vi "gmmregRegistrationTestNew.vi"() -> ()   [LabVIEW 2017]
panel:
  out "optogenetics (scene)":dbl[][](array[numeric])
  out "XY Graph 4":cluster{dbl[], dbl[]}[](graph)
  out "XY Graph 3":cluster{dbl[], dbl[]}(graph)
  out "XY Graph 2":cluster{dbl[], dbl[]}[](graph)
  out "XY Graph":cluster{dbl[], dbl[]}(graph)
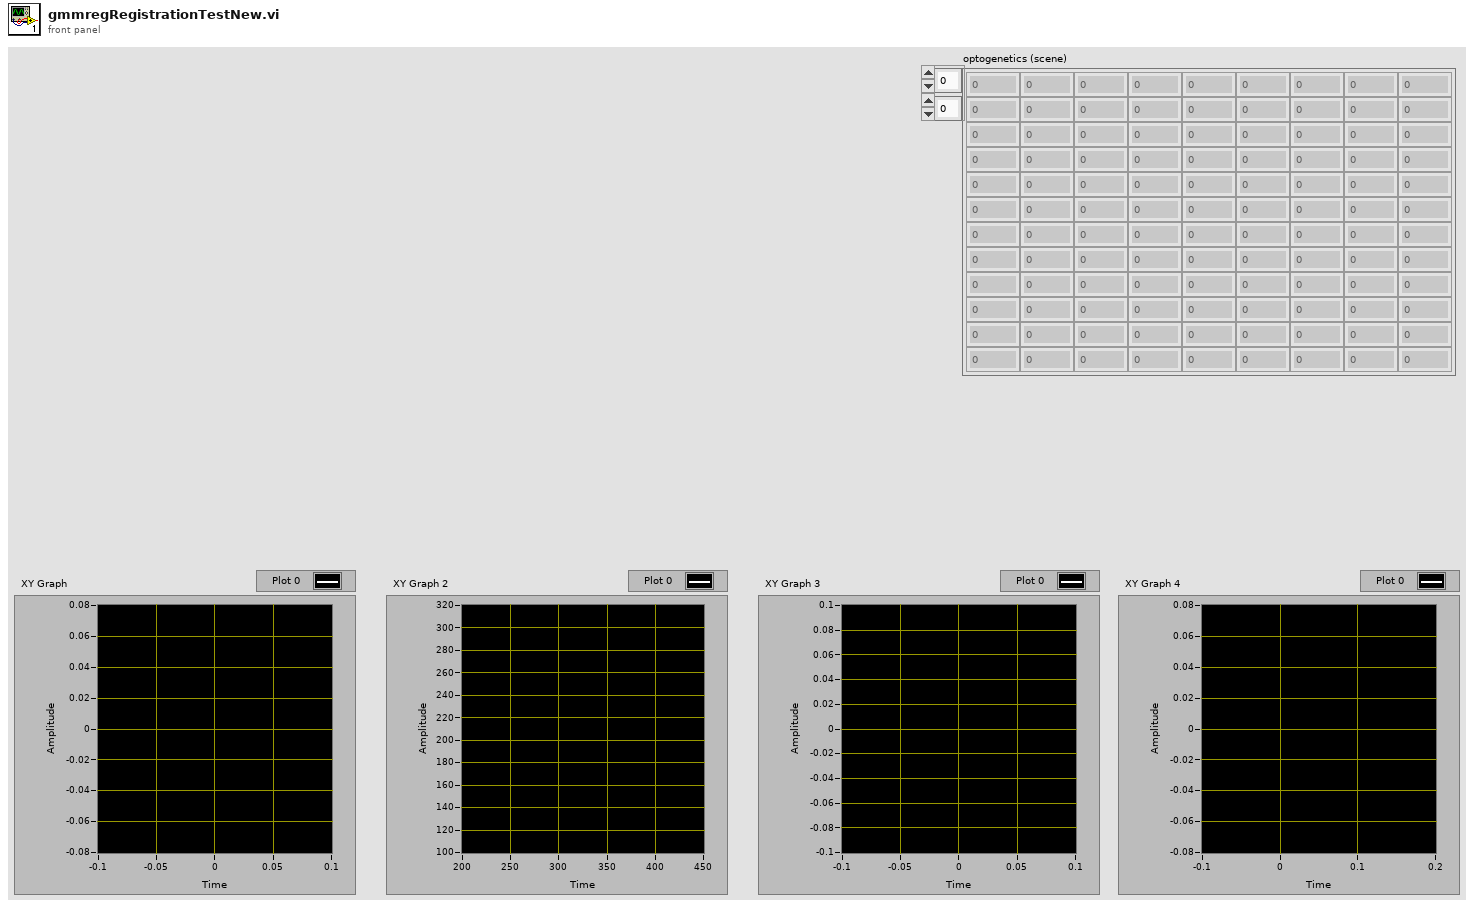
[diagram p1: front panel]
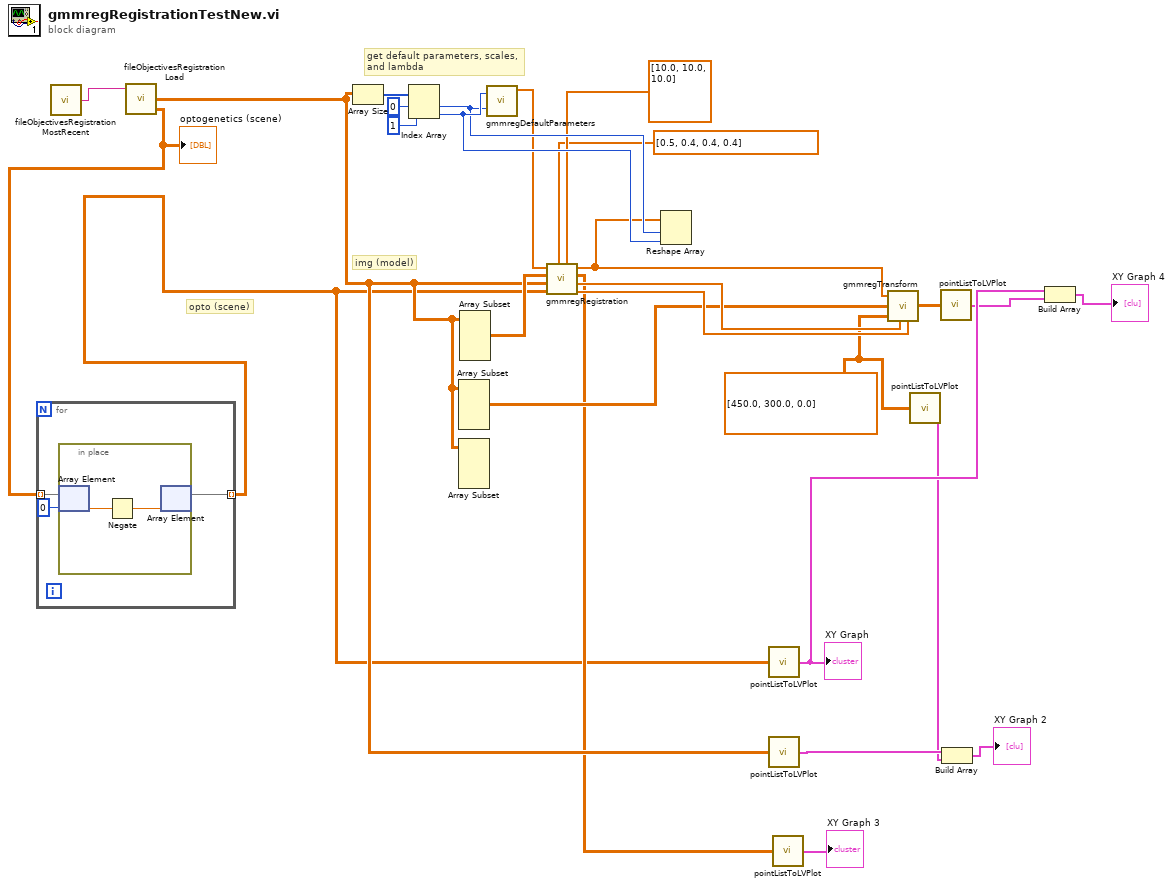
[diagram p0: block diagram]
diagram:
  w3 = dbl[][] [[450.0, 300.0, 0.0]] ("pts")
  # "get default parameters, scales,\nand lambda"
  # "img (model)"
  # "opto (scene)"
  n1 = call "fileObjectivesRegistrationMostRecent.vi"() -> ("f"=w27:string)  [unwired: 1 in]
  n2 = call "fileObjectivesRegistrationLoad.vi"("objectiveRegistrationFilePath"=w27) -> ("imaging (model)"=w15:dbl[][], "optogenetics (scene)"=w2:dbl[][])  [unwired: 3 in, 4 out]
  "optogenetics (scene)" <- w2
  n3 = for {
    tunnel: w2 -> [w30] mode=indexing
    tunnel: [w28] -> w1 mode=indexing
    n4 = in-place {
      n5 = in-place-array #1(w30, 0) -> (w32:dbl)
      n6 = Negate(x=w32) -> (-x=w31:dbl)
      n7 = in-place-array #1(w31) -> (w28:dbl[])  [unwired: 1 out]
    }
  }
  n8 = Array Size(array=w15) -> (size(s)=w23:i32[])
  n9 = Index Array(array=w23, index #1=0 ("index"), index #2=1 ("index")) -> (element #1=w25:i32, element #2=w26:i32)
  n10 = Array Subset(array=w15) -> (w16:dbl[][])  [unwired: 4 in]
  n11 = Array Subset(array=w15) -> ()  [unwired: 4 in, 1 out]
  n12 = Array Subset(array=w15) -> (w17:dbl[][])  [unwired: 4 in]
  n13 = call "gmmregDefaultParameters.vi"("D (3)"=w26, "nctrlPts"=w25) -> ("param0"=w24:dbl[])  [unwired: 3 out]
  n14 = call "gmmregRegistration.vi"("lambda"=dbl[] [10.0, 10.0, 10.0], "scale"=dbl[] [0.5, 0.4, 0.4, 0.4], "scene"=w1, "model"=w15, "ctrlPoints"=w17, "param0"=w24) -> ("denormParams out"=w18:dbl[], "normParams out"=w19:dbl[], "out"=w14:dbl[][], "param0 out"=w20:dbl[])  [unwired: 2 in]
  n15 = Reshape Array(w20, w25, w26) -> ()  [unwired: 1 out]
  n16 = call "pointListToLVPlot.vi"("XY[N,d]"=w1) -> ("LV plot"=w10:cluster{dbl[], dbl[]})
  "XY Graph" <- w10
  n17 = call "pointListToLVPlot.vi"("XY[N,d]"=w15) -> ("LV plot"=w7:cluster{dbl[], dbl[]})
  n18 = call "pointListToLVPlot.vi"("XY[N,d]"=w14) -> ("LV plot"=→"XY Graph 3":cluster{dbl[], dbl[]})
  n19 = call "gmmregTransform.vi"("param0"=w20, "ctrlPts"=w16, "pts"=w3, "normParams"=w19, "denormParams"=w18) -> ("out"=w12:dbl[][])  [unwired: 4 in]
  n20 = call "pointListToLVPlot.vi"("XY[N,d]"=w3) -> ("LV plot"=w6:cluster{dbl[], dbl[]})
  n21 = call "pointListToLVPlot.vi"("XY[N,d]"=w12) -> ("LV plot"=w9:cluster{dbl[], dbl[]})
  n22 = Build Array(w7, w6) -> (→"XY Graph 2":cluster{dbl[], dbl[]}[])
  n23 = Build Array(w10, w9) -> (→"XY Graph 4":cluster{dbl[], dbl[]}[])
